vi "BP.vi"() -> ()   [LabVIEW 2019, in "GUI Test HIPRESS.lvclass"]
uses:
  GUI Test HIPRESS.lvclass
panel:
  out "30":bool
  out "33.7 2":bool
  out "41.2":dbl
  out "41.1":dbl
  out "38.1":dbl
  out "Statte oil Supply 2":string="Состояние: Включенна" caption="НС Очистки и охлаждения"
  out "5.1":dbl
  out "4.1":dbl
  out "5.2":dbl
  out "4.2":dbl
  out "Statte oil Supply":string="Состояние: Включенна" caption="НС Подачи масла"
  out "41.3":dbl
  out "44.1":bool
  out "44.2":bool
  out "37.3":bool
  out "37.1":bool
  out "33.6":bool
  out "38.3":dbl
  out "38.2":dbl
  out "33.4":bool
  out "33.5":bool
  out "33.10":bool
  out "33.11":bool
  out "33.9":bool
  out "33.12":bool
  out "33.13":bool
  out "33.3":bool
  out "33.8":bool
  out "33.2":bool
  out "33.1":bool
  out "33.7":bool
  # "Камера"
  # "Образец"
  # "42"
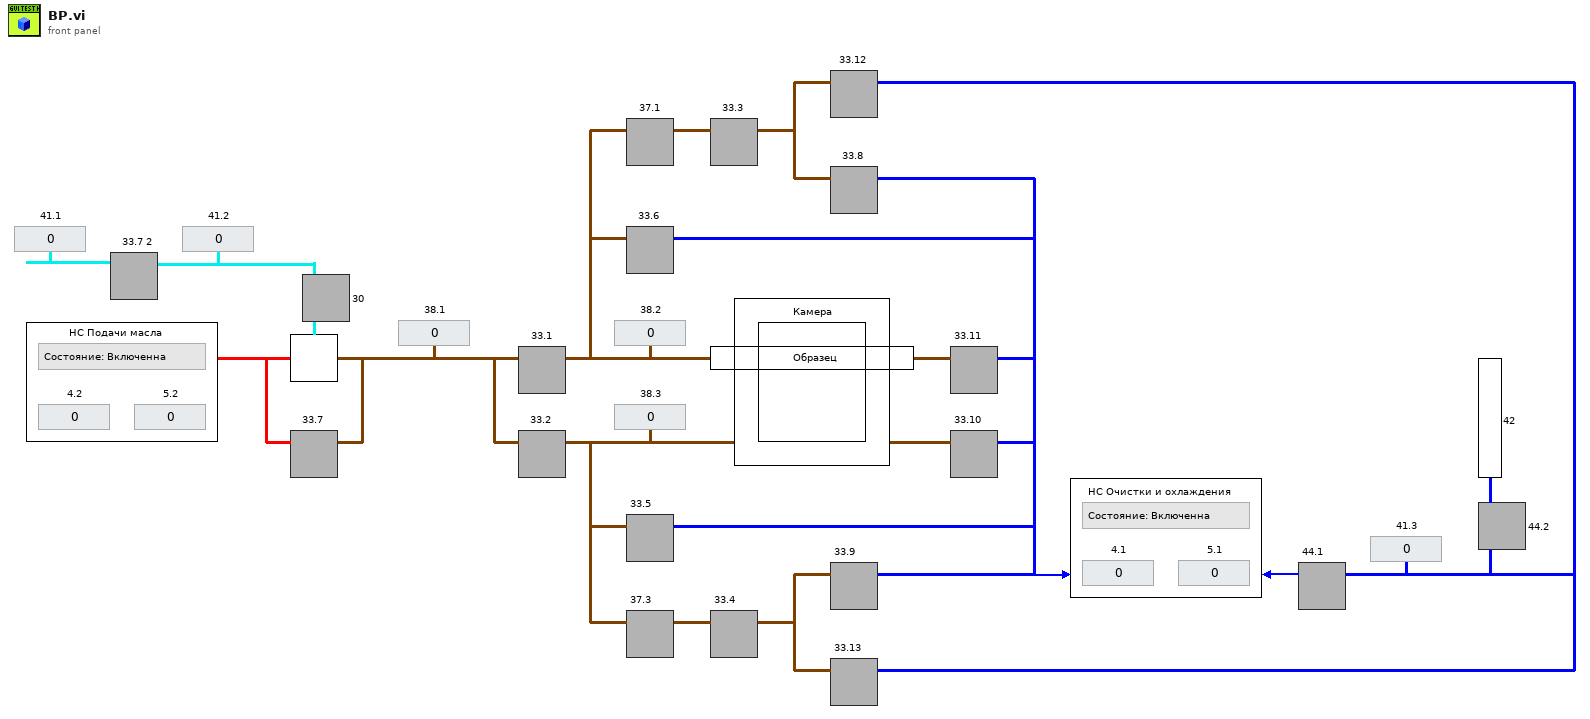
[diagram p1: front panel]
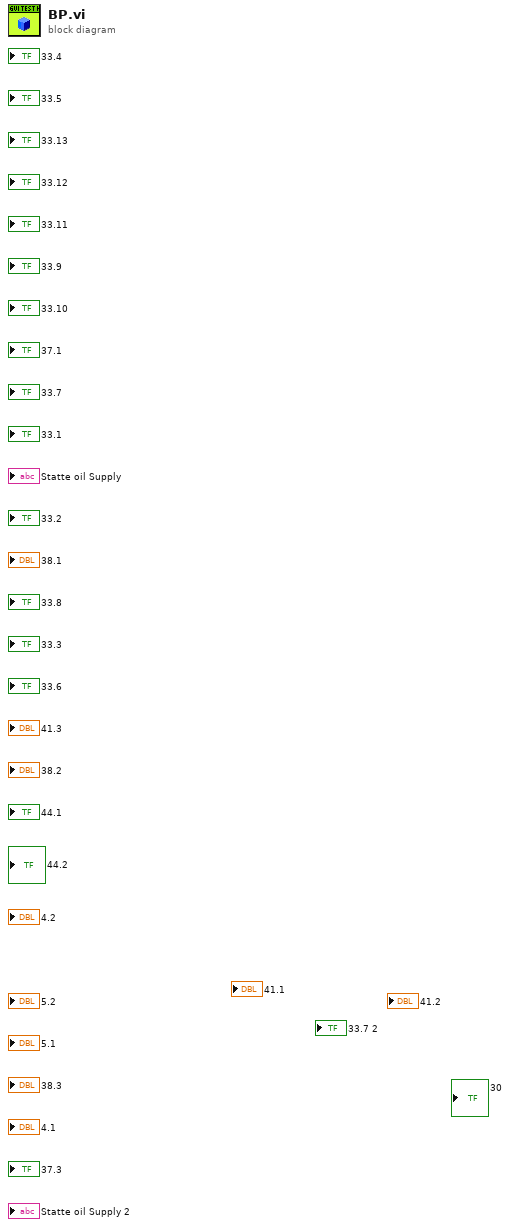
[diagram p0: block diagram]
diagram:
